vi "Revision Query.vi"(8 "error in (no error)":errorcluster, 11 "VISA resource name":refnum<visa-resource-name>) -> (0 "error out":errorcluster, 1 "Instrument Firmware Revision":string, 2 "Instrument Driver Revision":string, 3 "VISA resource name out":refnum<visa-resource-name>)   [LabVIEW 2013, in "HadCon.lvlib"]
doc: "Queries the current instrument firmware revision and instrument driver revision.\n\nRefer to the Readme file for detailed driver information including modification history."
uses:
  <instrlib>/HadCon/HadCon.lvlib
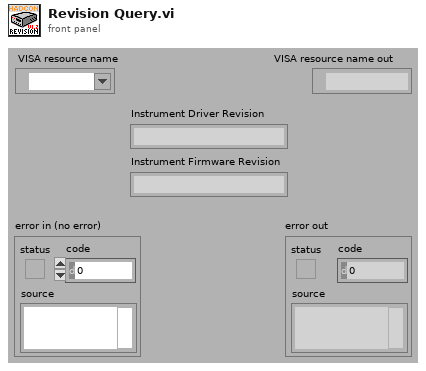
[diagram p1: front panel]
types:
  T1 = cluster{"Major":u16, "Minor":u16, "Fix":u16, "Build":u16}
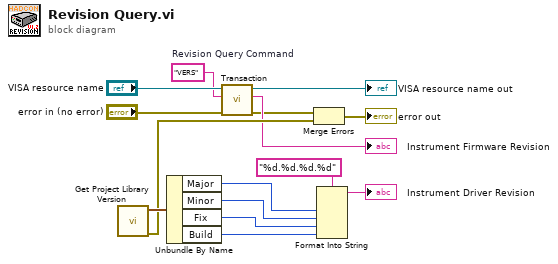
[diagram p0: block diagram]
diagram:
  w10 = "VERS"  # Revision Query Command
  n1 = call <vilib>:"Get Project Library Version.vi"() -> ("error out"=w8:errorcluster, "Project Library Version"=w12:T1)  [unwired: 10 in]
  n2 = Unbundle By Name(w12) -> ("Major"=w14:u16, "Minor"=w13:u16, "Fix"=w6:u16, "Build"=w5:u16)
  n3 = call <instrlib>:"Transaction.vi"("Error In"="error in (no error)", "Command"=w10, "VISA resource name"="VISA resource name") -> ("Error Out"=w2:errorcluster, "Response"=→"Instrument Firmware Revision":string, "VISA resource name out"=→"VISA resource name out":refnum<visa-resource-name>)  [unwired: 6 in]
  n4 = Merge Errors(w2, w8) -> (→"error out":errorcluster)
  n5 = Format Into String(format string="%d.%d.%d.%d", w14, w13, w6, w5) -> (resulting string=→"Instrument Driver Revision":string)  [unwired: 2 in, 1 out]
